vi "_Read Buffer No Objects - Photon Counter.vi"(7 "Photon Counter SR 400 in":T1={"Mode"=0, "Count Time"=0.0, "Trigger Frequency"=10000000.0, "Trigger External?"=FALSE, "Gate A Mode"=0, "Gate A Width"=0.0, "Gate A Delay"=0.0, "Gate B Mode"=0, "Gate B Width"=0.0, "Gate B Delay"=0.0} {"Mode" items=["A,B For T Preset", "A-B For T Preset", "A+B For T Preset", "A For B Preset"]; "Gate A Mode" items=["CW", "Fixed"]; "Gate B Mode" items=["CW", "Fixed"]}, 8 "error in (no error)":errorcluster, 11 "VISA Resource Name In":refnum<visa-resource-name>="GPIB0::23::INSTR") -> (0 "error out":errorcluster, 1 "appended array":dbl[](array[numeric]), 3 "VISA Resource Name Out":refnum<visa-resource-name>="GPIB0::23::INSTR", 5 "Photon Counter SR 400 out":T1={"Mode"=0, "Count Time"=0.0, "Trigger Frequency"=10000000.0, "Trigger External?"=FALSE, "Gate A Mode"=0, "Gate A Width"=0.0, "Gate A Delay"=0.0, "Gate B Mode"=0, "Gate B Width"=0.0, "Gate B Delay"=0.0} {"Mode" items=["A,B For T Preset", "A-B For T Preset", "A+B For T Preset", "A For B Preset"]; "Gate A Mode" items=["CW", "Fixed"]; "Gate B Mode" items=["CW", "Fixed"]})   [LabVIEW 2015]
uses:
  SR400.lvlib
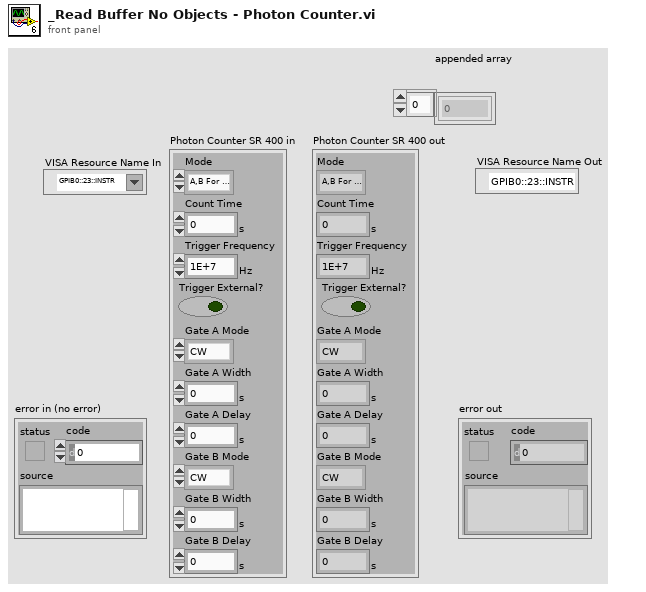
[diagram p1: front panel]
types:
  T1 = cluster{"Mode":u16, "Count Time":dbl[unit], "Trigger Frequency":dbl[unit], "Trigger External?":bool, "Gate A Mode":u16, "Gate A Width":dbl[unit], "Gate A Delay":dbl[unit], "Gate B Mode":u16, "Gate B Width":dbl[unit], "Gate B Delay":dbl[unit]}
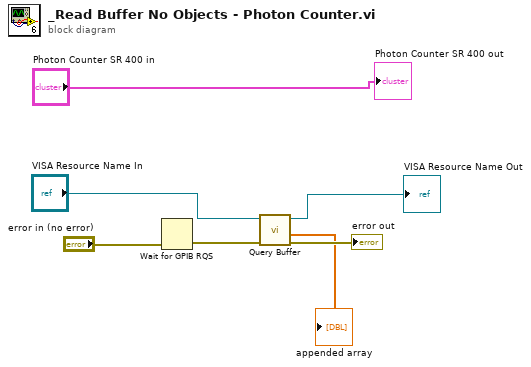
[diagram p0: block diagram]
diagram:
  n1 = Wait for GPIB RQS(2:"error in (no error)") -> (0:w2:errorcluster)  [unwired: 2 in, 1 out]
  n2 = call "Query Buffer.vi"("error in (no error)"=w2, "VISA resource name"="VISA Resource Name In") -> ("error out"=→"error out":errorcluster, "appended array"=→"appended array":dbl[], "VISA resource name out"=→"VISA Resource Name Out":refnum<visa-resource-name>)  [unwired: 7 in]
  "Photon Counter SR 400 out" <- "Photon Counter SR 400 in"
